vi "Bilinear Prewarping of f.vi"(1 "freq specs [Hz]":T1) -> (0 "prewarped freq specs [Hz]":T1)   [LabVIEW 2020, in "NI_AAL_Filter.lvlib"]
uses:
  <vilib>/Analysis/NI_AAL_Filter.lvlib
  <vilib>/Analysis/3filter.llb/Filter Frequence Specification (Design).ctl
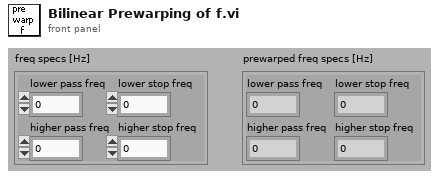
[diagram p1: front panel]
types:
  T1 = typedef "NI_AAL_Filter.lvlib/Filter Frequence Specification (Design).ctl" = cluster{"lower pass freq":dbl, "lower stop freq":dbl, "higher pass freq":dbl, "higher stop freq":dbl}
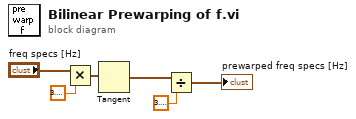
[diagram p0: block diagram]
diagram:
  n1 = Multiply(x="freq specs [Hz]", y=3.141592653589793) -> (x*y=w6:T1)
  n2 = Tangent(1:w6) -> (0:w3:T1)
  n3 = Divide(x=w3, y=3.141592653589793) -> (x/y=→"prewarped freq specs [Hz]":T1)
